vi "Initialize.vi"(8 "error in (no error)":errorcluster, 10 "Microscope Configuration":T1={"Serial Port"="COM2", "Microscope Type"=enum."TE2000", "Detection Settings"=[]}, 11 "Nikon Stand in":refnum<class "Nikon Stand.lvclass">) -> (0 "error out":errorcluster, 3 "Nikon Stand out":refnum<class "Nikon Stand.lvclass">)   [LabVIEW 2023, in "Nikon Stand.lvlib" / "Nikon Stand.lvclass"]
uses:
  Nikon Stand.lvclass
  Resources/Type Defs/Microscope Configuration.ctl
  Resources/Type Defs/Microscope Type.ctl
  Nikon Stand.lvclass/Nikon Stand.ctl
  Microscope/ti2lv/ti2lv.lvlib
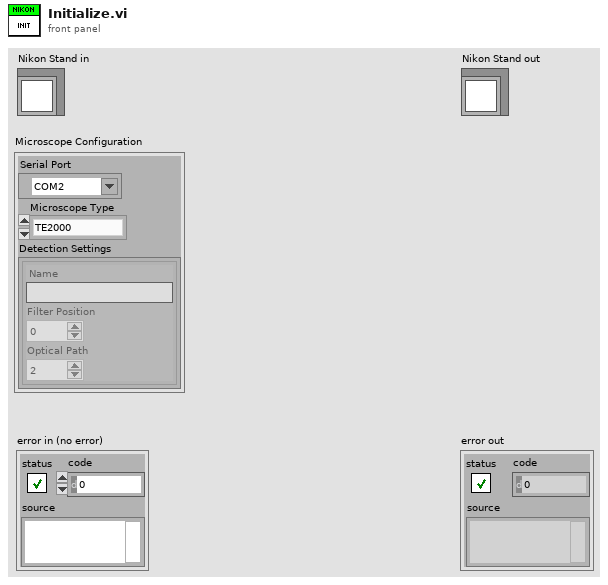
[diagram p1: front panel]
types:
  T1 = typedef "Microscope Configuration.ctl" = cluster{"Serial Port":refnum<visa-resource-name>, "Microscope Type":T2, "Detection Settings":cluster{"Name":string, "Filter Position":u16, "Optical Path":u16}[]}
  T2 = typedef "Microscope Type.ctl" = enum16{"Disable", "TE2000", "Eclipse Ti", "Ti2"}
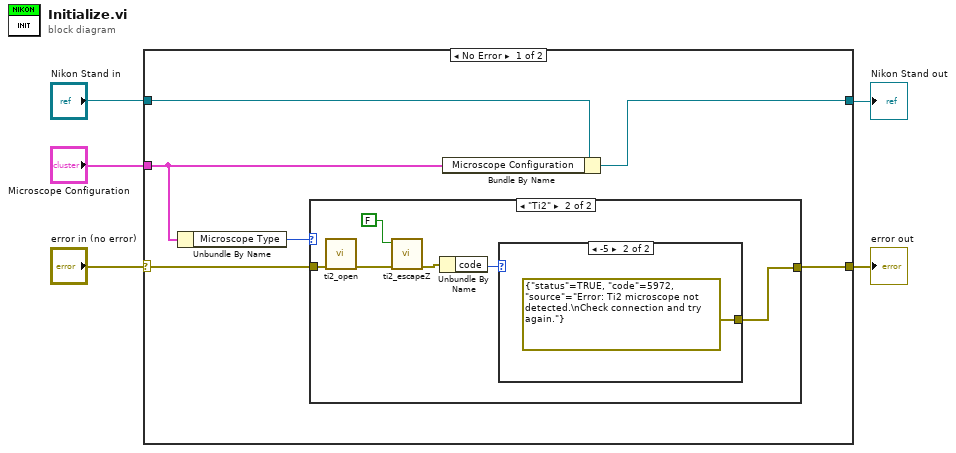
[diagram p0: block diagram]
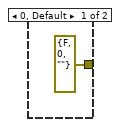
[diagram p3: hidden frame]
diagram:
  n1 = case shown="No Error" "error in (no error)" {
    selector: "error in (no error)" -> [w11 w22]
    tunnel: [w8 w22] -> w2
    tunnel: "Nikon Stand in" -> [w10 w21]
    tunnel: [w9 w21] -> w1
    tunnel: "Microscope Configuration" -> [w7 _]
    frame No Error {
      n2 = Unbundle By Name(w7) -> ("Microscope Type"=w6:T2)
      n3 = case shown="\"Ti2\"" w6 {
        tunnel: w11 -> [w12 w17]
        tunnel: [w12 w16] -> w8
        frame "Disable", Default {
        }
        frame "Ti2" {
          n4 = call "ti2_open.vi"("error in (no error)"=w17) -> ("error out"=w14:errorcluster)  [unwired: 10 in]
          n5 = call "ti2_escapeZ.vi"("error in (no error)"=w14, "Escape Z"=FALSE) -> ("error out"=w13:errorcluster)  [unwired: 9 in]
          n6 = Unbundle By Name(w13) -> ("code"=w18:i32)
          n7 = case shown="-5" w18 {
            tunnel: [errorcluster {"status"=FALSE, "code"=0, "source"=""} ("error constant") errorcluster {"status"=TRUE, "code"=5972, "source"="Error: Ti2 microscope not detected.\nCheck connection and try again."} ("error constant")] -> w16
            frame 0, Default {
            }
            frame -5 {
            }
          }
        }
      }
      n8 = Bundle By Name(cluster=w10, "Microscope Configuration"=w7) -> (w9:refnum<class "Nikon Stand.lvclass">)
    }
    frame Error {
    }
  }
  "error out" <- w2
  "Nikon Stand out" <- w1
